vi "Copy Data.vi"   [LabVIEW 2013, in "main.lvlib"]
uses:
  main.lvlib
  <userlib>/_OpenG.lib/file/file.llb/File Exists - Scalar__ogtk.vi
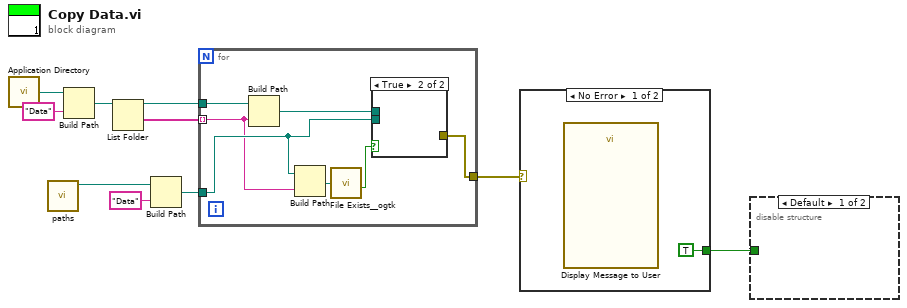
[diagram p0: block diagram]
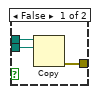
[diagram p2: hidden frame]
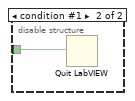
[diagram p3: hidden frame]
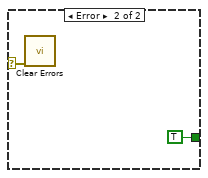
[diagram p4: hidden frame]
diagram:
  n1 = call <vilib>:"Application Directory.vi"() -> ("Application Directory"=w10:path)
  n2 = call "paths.vi"() -> ("PubAppData"=w6:path)  [unwired: 8 in, 3 out]
  n3 = Build Path(base path=w10, name or relative path="Data") -> (appended path=w2:path)
  n4 = List Folder(path=w2) -> (path out=w3:path, folder names=w1:string[])  [unwired: 3 in, 2 out]
  n5 = Build Path(base path=w6, name or relative path="Data") -> (appended path=w4:path)
  n6 = for {
    tunnel: [w15] -> w7
    tunnel: w4 -> [w14]
    tunnel: w3 -> [w17]
    tunnel: w1 -> [w13] mode=indexing
    n7 = Build Path(base path=w17, name or relative path=w13) -> (appended path=w16:path)
    n8 = Build Path(base path=w14, name or relative path=w13) -> (appended path=w12:path)
    n9 = call-poly <userlib>:"File Exists__ogtk.vi"("file path"=w12) -> ("exists"=w11:bool)  [unwired: 6 in, 1 out]
    n10 = case shown="True" w11 {
      tunnel: w16 -> [w20 _]
      tunnel: [w19 _] -> w15
      tunnel: w14 -> [w18 _]
      frame False {
        n11 = Copy(10:w18, 11:w20) -> (0:w19:errorcluster)  [unwired: 3 in, 2 out]
      }
      frame True {
      }
    }
  }
  n12 = case shown="No Error" w7 {
    selector: w7 -> [_ w22]
    tunnel: [TRUE ("Close") TRUE ("Close")] -> w8
    frame No Error {
      n13 = call "Display Message to User"() -> ()  [unwired: 10 in, 2 out]
    }
    frame Error {
      n14 = call <vilib>:"Clear Errors.vi"("error in (no error)"=w22) -> ()  [unwired: 6 in, 1 out]
    }
  }
  n15 = disable-structure shown="Default" {
    disable-tunnel: w8 -> [_ w24]
    frame condition #0 (active) {
    }
    frame condition #1 {
      n16 = Quit LabVIEW(quit? (T)=w24) -> ()
    }
  }
